vi "AttrMap-GetValue2.vi"(8 "error in (no error)":errorcluster, 9 "Key":string, 11 "AttrMap in":T1) -> (0 "error out":errorcluster, 2 "data":variant, 3 "AttrMap out":T1, 4 "OrignKey":string)   [LabVIEW 2019, in "lv-apt-json-file.lvlib"]
uses:
  lv-apt-json-file.lvlib
  Typedef/Def-AttrMap.ctl
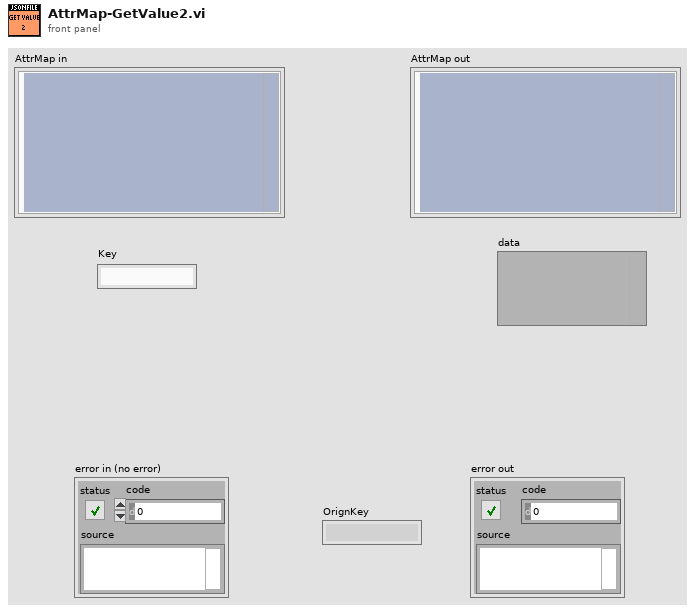
[diagram p1: front panel]
types:
  T1 = typedef "lv-apt-json-file.lvlib/Def-AttrMap.ctl" = cluster{"Map":variant}
  T2 = typedef "lv-apt-json-file.lvlib/Def-AttrMap -- Map.ctl" = map{string, string}
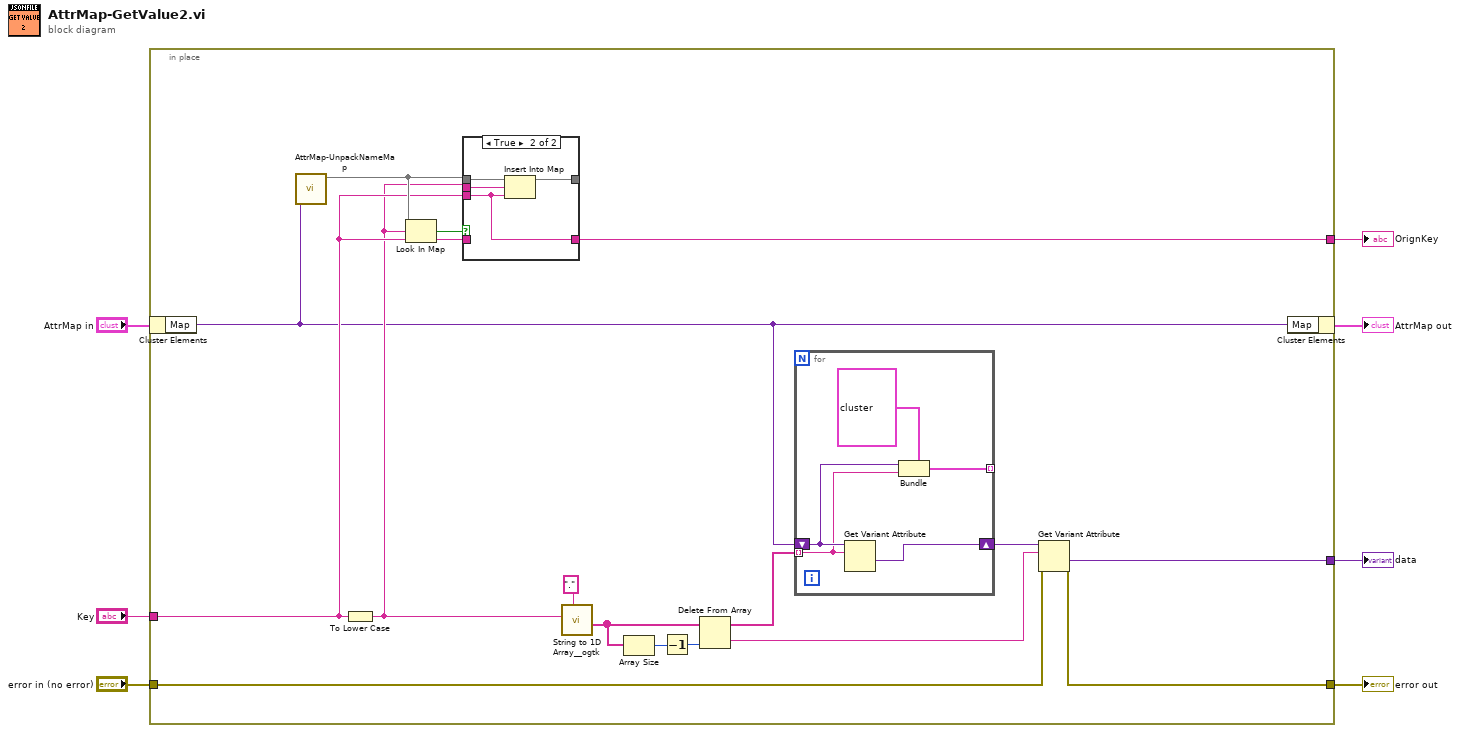
[diagram p0: block diagram]
diagram:
  n1 = in-place {
    in-place-border: [w23] -> w7
    in-place-border: "error in (no error)" -> [w24]
    in-place-border: "Key" -> [w19]
    in-place-border: [w9] -> w2
    in-place-border: [w8] -> w1
    n2 = in-place-cluster #1("AttrMap in") -> ("Map"=w10:variant)
    n3 = call "AttrMap-UnpackNameMap.vi"("Map"=w10) -> ("NameMap"=w20:T2)  [unwired: 10 in]
    n4 = To Lower Case(string=w19) -> (all lower case string=w16:string)
    n5 = Look In Map(map=w20, key=w16, default value=w19) -> (key not found?=w22:bool, value=w21:string)
    n6 = case shown="True" w22 {
      tunnel: w20 -> [w31 w35]
      tunnel: [w31 w34] -> _
      tunnel: w16 -> [_ w33]
      tunnel: w19 -> [_ w32]
      tunnel: w21 -> [w30 _]
      tunnel: [w30 w32] -> w8
      frame False {
      }
      frame True {
        n7 = Insert Into Map(map in=w35, key=w33, value=w32) -> (map out=w34:T2)  [unwired: 2 out]
      }
    }
    n8 = call <userlib>:"String to 1D Array__ogtk.vi"("delimiter (Tab)"=".", "string"=w16) -> ("Array of Strings"=w13:string[])  [unwired: 9 in]
    n9 = Array Size(array=w13) -> (size(s)=w17:i32)
    n10 = Decrement(x=w17) -> (x-1=w11:i32)
    n11 = Delete From Array(array=w13, index=w11) -> (deleted portion=w14:string, array with subset deleted=w12:string[])  [unwired: 1 in]
    n12 = for {
      tunnel: w12 -> [w28] mode=indexing
      shift-right: [w27] -> w15
      shift-left: w10 -> [w29]
      tunnel: [w25] -> _ mode=indexing
      n13 = Get Variant Attribute(Variant=w29, name=w28) -> (value=w27:variant)  [unwired: 2 in, 3 out]
      n14 = Bundle(cluster=cluster{"Parent":variant, "Name":string} {"Parent"=variant, "Name"=""}, "Parent"=w29, "Name"=w28) -> (w25:cluster{"Parent":variant, "Name":string})
    }
    n15 = Get Variant Attribute(Variant=w15, name=w14, error in=w24) -> (value=w9:variant, error out=w23:errorcluster)  [unwired: 1 in, 2 out]
    n16 = in-place-cluster #1("Map"=w10) -> (→"AttrMap out":T1)
  }
  "error out" <- w7
  "data" <- w2
  "OrignKey" <- w1
